vi "act-cor.vi"() -> ()   [LabVIEW 2010]
panel:
  in  "options":i32
  in  "chemin du VI":path
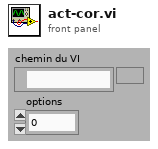
[diagram p1: front panel]
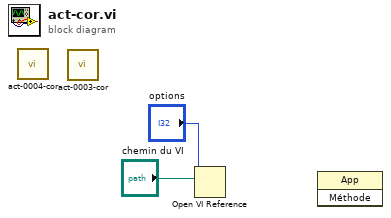
[diagram p0: block diagram]
diagram:
  n1 = call "act-0004-cor.vi"() -> ()  [unwired: 1 in, 1 out]
  n2 = call "act-0003-cor.vi"() -> ()  [unwired: 12 in]
  n3 = Open VI Reference(vi path="chemin du VI", options="options") -> ()  [unwired: 4 in, 2 out]
  n4 = invoke class="App" method=#-1() -> ()  [unwired: 3 in, 3 out]
